vi "removeConnection.vi"(8 "error in (no error) 2":errorcluster, 9 "conection id (string)":string, 10 "variable(s)":string, 11 "variable variant in":variant) -> (0 "error out":errorcluster, 3 "variable variant out":variant)   [LabVIEW 2011]
uses:
  variabledata_typdef.ctl
panel:
  out "format string":string
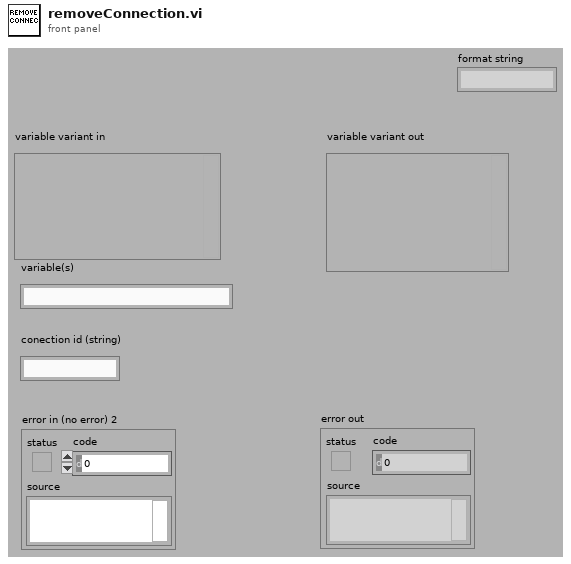
[diagram p1: front panel]
types:
  T1 = typedef "variabledata_typdef.ctl" = cluster{"type":string, "connections (ID)":string, "compressed":bool, "non compressed":bool}
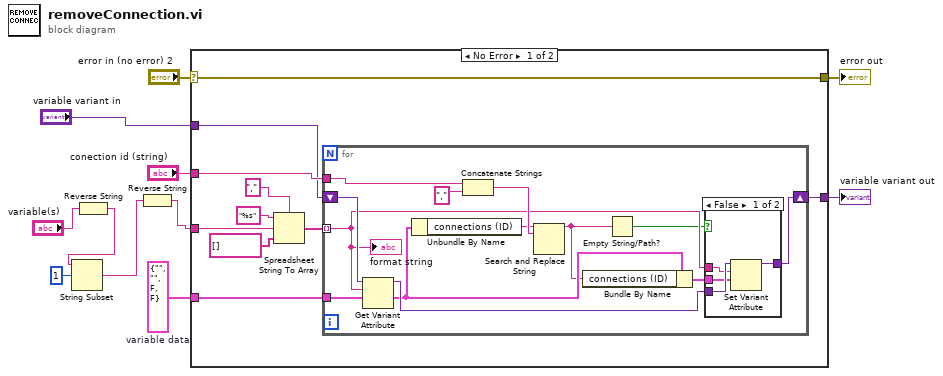
[diagram p0: block diagram]
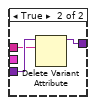
[diagram p2: hidden frame]
diagram:
  w6 = T1 {"type"="", "connections (ID)"="", "compressed"=FALSE, "non compressed"=FALSE}  # variable data
  n1 = Reverse String(1:"variable(s)") -> (0:w3:string)
  n2 = String Subset(string=w3, offset (0)=1) -> (substring=w2:string)  [unwired: 1 in]
  n3 = Reverse String(1:w2) -> (0:w1:string)
  n4 = case shown="No Error" "error in (no error) 2" {
    selector: "error in (no error) 2" -> [w15 w42]
    tunnel: "conection id (string)" -> [w21 _]
    tunnel: "variable variant in" -> [w20 w43]
    tunnel: w1 -> [w13 _]
    tunnel: [w16 w43] -> w9
    tunnel: [w15 w42] -> w11
    tunnel: w6 -> [w14 _]
    frame No Error {
      n5 = Spreadsheet String To Array(delimiter (Tab)="," ("format string"), format string="%s", spreadsheet string=w13, array type (2D Dbl)=string[] []) -> (array=w12:string[])
      n6 = for {
        tunnel: w12 -> [w28] mode=indexing
        tunnel: w21 -> [w31]
        shift-right: [w33] -> w16
        shift-left: w20 -> [w32]
        tunnel: w14 -> [w26]
        n7 = Get Variant Attribute(Variant=w32, name=w28, default value (empty Variant)=w26) -> (duplicate Variant=w34:variant, value=w24:T1)  [unwired: 1 in, 2 out]
        n8 = Unbundle By Name(w24) -> ("connections (ID)"=w25:string)
        n9 = Concatenate Strings(w31, "," ("string")) -> (w29:string)
        n10 = Search and Replace String(input string=w25, search string=w29) -> (result string=w23:string)  [unwired: 6 in, 3 out]
        n11 = Bundle By Name(cluster=w24, "connections (ID)"=w23) -> (w22:T1)
        n12 = Empty String/Path?(string/path=w23) -> (empty?=w27:bool)
        n13 = case shown="False" w27 {
          tunnel: w34 -> [w38 w41]
          tunnel: [w37 w40] -> w33
          tunnel: w28 -> [w36 w39]
          tunnel: w22 -> [w35 _]
          frame False {
            n14 = Set Variant Attribute(Variant=w38, name=w36, value=w35) -> (Variant out=w37:variant)  [unwired: 1 in, 2 out]
          }
          frame True {
            n15 = Delete Variant Attribute(6:w39, 7:w41) -> (3:w40:variant)  [unwired: 1 in, 2 out]
          }
        }
        "format string" <- w28
      }
    }
    frame Error {
    }
  }
  "variable variant out" <- w9
  "error out" <- w11
